vi "SetSpeed.vi"(8 "error in (no error)":errorcluster, 10 "Speed(0..4095)":u16, 11 "DCMotor in":refnum<class "DCMotor.lvclass">) -> (0 "error out":errorcluster, 3 "DCMotor out":refnum<class "DCMotor.lvclass">)   [LabVIEW 2022 SP3, in "Motorshield.lvlib" / "DCMotor.lvclass"]
uses:
  DCMotor.lvclass
  C:/Users/Carlos/Desktop/onlab/source/Motorshield/Motorshield/Motorshield.lvclass
  DCMotor.lvclass/DCMotor.ctl
  Motorshield/Motorshield.lvclass
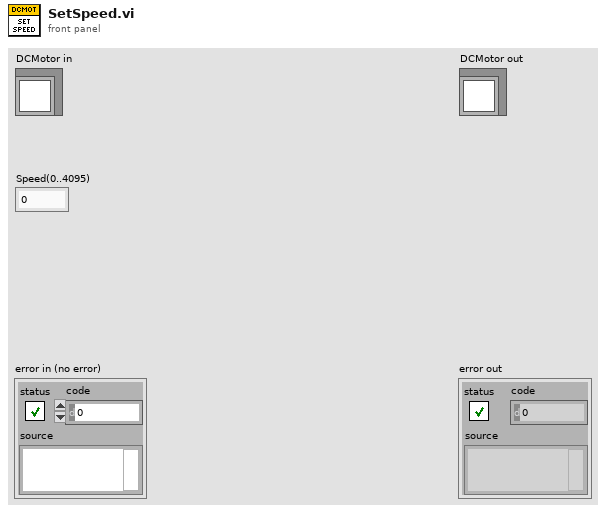
[diagram p1: front panel]
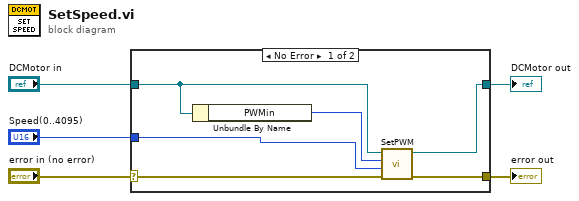
[diagram p0: block diagram]
diagram:
  n1 = case shown="No Error" "error in (no error)" {
    selector: "error in (no error)" -> [w11 w13]
    tunnel: [w10 w13] -> w4
    tunnel: [w9 w12] -> w2
    tunnel: "DCMotor in" -> [w8 w12]
    tunnel: "Speed(0..4095)" -> [w6 _]
    frame No Error {
      n2 = Unbundle By Name(w8) -> ("PWMin"=w7:u8)
      n3 = call "SetPWM.vi"("error in (no error)"=w11, "Value"=w6, "Led num"=w7, "Motorshield in"=w8) -> ("error out"=w10:errorcluster, "Motorshield out"=w9:refnum<class "DCMotor.lvclass">)  [unwired: 6 in]
    }
    frame Error {
    }
  }
  "error out" <- w4
  "DCMotor out" <- w2
